vi "Read.vi"(8 "error in (no error)":errorcluster, 11 "Boolean in":refnum<class "OnChangeNotifier_DBL.lvclass">) -> (0 "error out":errorcluster, 2 "Value":T1, 3 "Boolean out":refnum<class "OnChangeNotifier_DBL.lvclass">)   [LabVIEW 2021, in "OnChangeNotifier_DBL.lvclass"]
doc: "Abstract Data Classes 2.1.1.13\nTim Streeter - TSA\nCopyright (c) 2025, TSA"
uses:
  OnChangeNotifier_DBL.lvclass
  OnChangeNotifier_DBL.lvclass/OnChangeNotifier_DBL.ctl
  <vilib>/TSA/Abstract Data Classes/Abs_Types/Single Float/Abs_Single Float.lvclass
  Support/Type.ctl
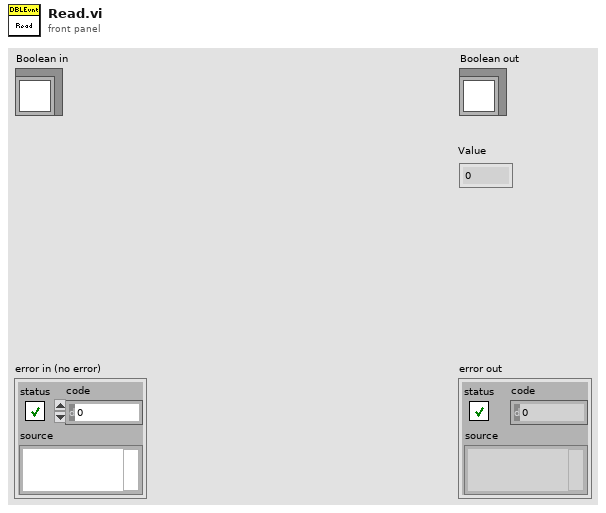
[diagram p1: front panel]
types:
  T1 = typedef "OnChangeNotifier_DBL.lvclass/Type.ctl" = sgl
  T2 = typedef "OnChangeNotifier_DBL.lvclass/Class Type.ctl" = refnum<class "Abs_Single Float.lvclass">
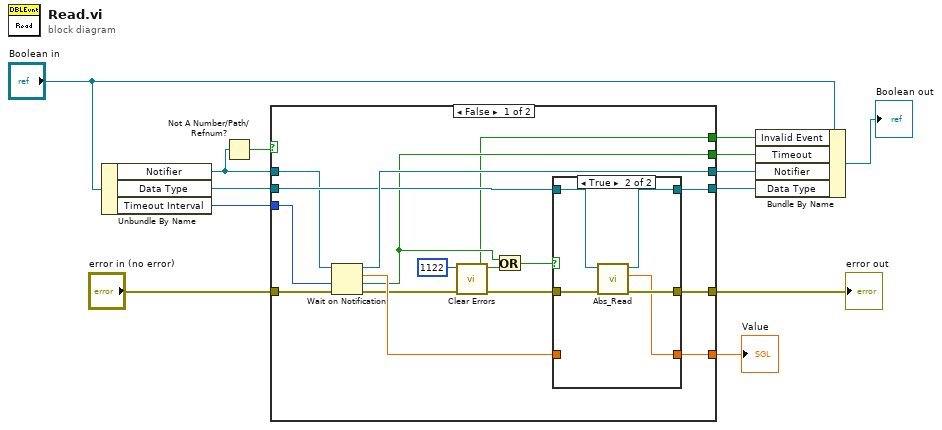
[diagram p0: block diagram]
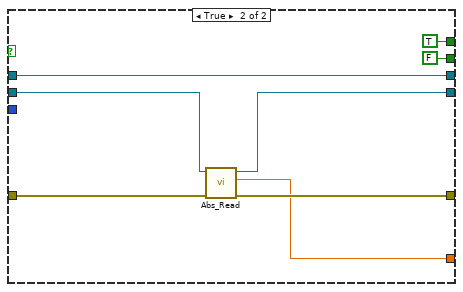
[diagram p3: hidden frame]
diagram:
  n1 = Unbundle By Name("Boolean in") -> ("Notifier"=w3:refnum<notifier>, "Data Type"=w8:T2, "Timeout Interval"=w6:i32)
  n2 = Not A Number/Path/Refnum?(number/path/refnum=w3) -> (NaN/Path/Refnum?=w2:bool)
  n3 = case shown="False" w2 {
    tunnel: [w28 w42] -> w12
    tunnel: "error in (no error)" -> [w27 w44]
    tunnel: [w26 w41] -> w10
    tunnel: [w25 w40] -> w9
    tunnel: w8 -> [w24 w43]
    tunnel: [w23 w39] -> w7
    tunnel: w6 -> [w22 _]
    tunnel: [w19 FALSE ("timed out?")] -> w5
    tunnel: [w17 TRUE ("specific error cleared?")] -> w4
    tunnel: w3 -> [w16 w42]
    frame False {
      n4 = Wait on Notification(notifier=w16, timeout in ms (-1)=w22, error in (no error)=w27) -> (notifier out=w28:refnum<notifier>, notification=w21:T1, timed out?=w19:bool, error out=w14:errorcluster)  [unwired: 1 in]
      n5 = call <vilib>:"Clear Errors.vi"("error in (no error)"=w14, "specific error code to clear (0: all)"=1122) -> ("error out"=w20:errorcluster, "specific error cleared?"=w17:bool)  [unwired: 4 in]
      n6 = Or(x=w19, y=w17) -> (x .or. y?=w18:bool)
      n7 = case shown="True" w18 {
        tunnel: w24 -> [w31 w36]
        tunnel: [w31 w35] -> w26
        tunnel: w20 -> [w30 w34]
        tunnel: [w30 w33] -> w25
        tunnel: [w29 w32] -> w23
        tunnel: w21 -> [w29 _]
        frame False {
        }
        frame True {
          # "Timeout"
          n8 = call-poly <vilib>:"Abs_Read.vi"("error in (no error)"=w34, "Abs_Single Float in"=w36) -> ("error out"=w33:errorcluster, "Value"=w32:sgl, "Abs_Single Float out"=w35:T2)  [unwired: 7 in]
        }
      }
    }
    frame True {
      n9 = call-poly <vilib>:"Abs_Read.vi"("error in (no error)"=w44, "Abs_Single Float in"=w43) -> ("error out"=w40:errorcluster, "Value"=w39:sgl, "Abs_Single Float out"=w41:T2)  [unwired: 7 in]
    }
  }
  "error out" <- w9
  "Value" <- w7
  n10 = Bundle By Name(cluster="Boolean in", "Invalid Event"=w4, "Timeout"=w5, "Notifier"=w12, "Data Type"=w10) -> (→"Boolean out":refnum<class "OnChangeNotifier_DBL.lvclass">)
